vi "Image Name.vi"(8 "error in (no error)":errorcluster, 11 "CCDCamera in":refnum<class "CCDCamera.lvclass">) -> (0 "error out":errorcluster, 3 "CCDCamera out":refnum<class "CCDCamera.lvclass">)   [LabVIEW 2018, in "CCDCamera.lvclass"]
uses:
  CCDCamera.lvclass
  CCDCamera.lvclass/CCDCamera.ctl
  Interface/Interface.lvclass
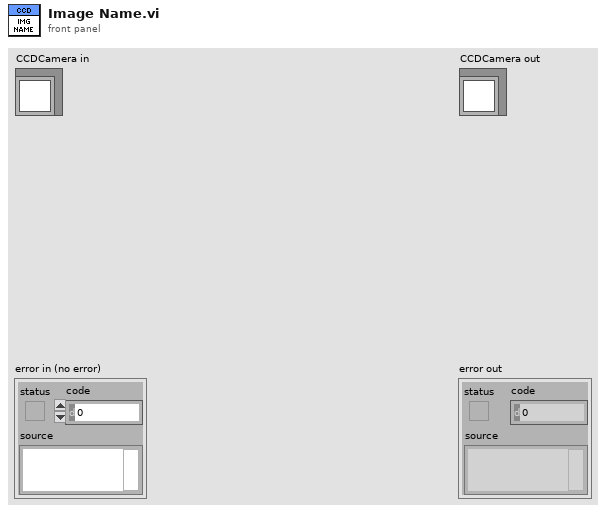
[diagram p1: front panel]
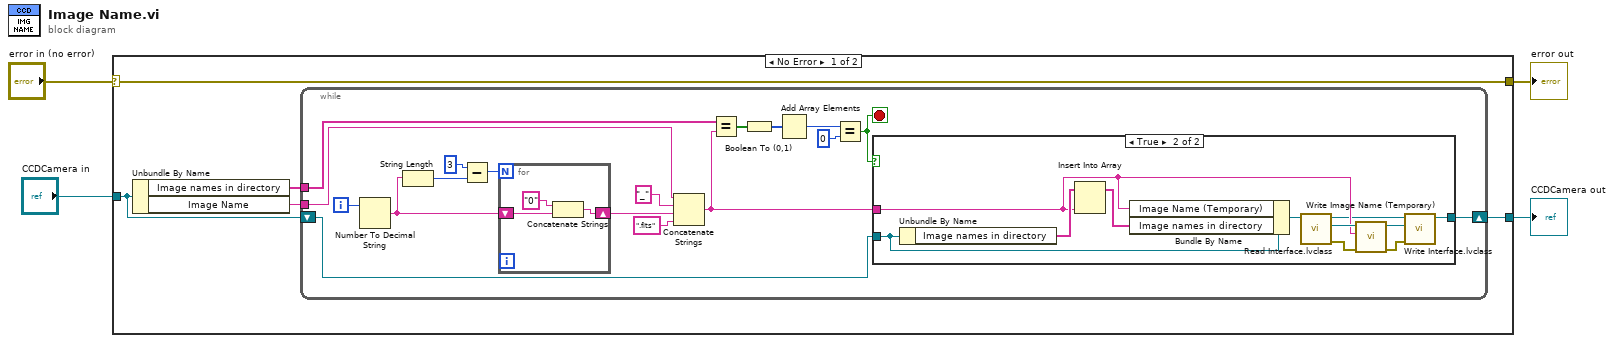
[diagram p0: block diagram]
diagram:
  n1 = case shown="No Error" "error in (no error)" {
    selector: "error in (no error)" -> [w9 w44]
    tunnel: [w9 w44] -> w3
    tunnel: [w7 w43] -> w1
    tunnel: "CCDCamera in" -> [w6 w43]
    frame No Error {
      n2 = Unbundle By Name(w6) -> ("Image names in directory"=w5:string[], "Image Name"=w8:string)
      n3 = while {
        tunnel: w5 -> [w27]
        tunnel: w8 -> [w19]
        shift-right: [w22] -> w7
        shift-left: w6 -> [w21]
        i -> [w20]
        stop <- w17 stop-if-true
        n4 = Number To Decimal String(number=w20) -> (decimal integer string=w10:string)  [unwired: 1 in]
        n5 = String Length(string=w10) -> (length=w13:i32)
        n6 = Subtract(x=3, y=w13) -> (x-y=w14:i32)
        n7 = for {
          N: w14 -> [_]
          shift-right: [w30] -> w11
          shift-left: w10 -> [w28]
          n8 = Concatenate Strings("0" ("string"), w28) -> (w30:string)
        }
        n9 = Concatenate Strings(w19, "_" ("string"), w11, ".fits" ("string")) -> (w18:string)
        n10 = Equal?(x=w27, y=w18) -> (x = y?=w26:bool[])
        n11 = Boolean To (0,1)(Boolean=w26) -> (0, 1=w25:i16[])
        n12 = Add Array Elements(numeric array=w25) -> (sum=w24:i16)
        n13 = Equal?(x=w24, y=0) -> (x = y?=w17:bool)
        n14 = case shown="True" w17 {
          tunnel: w18 -> [_ w33]
          tunnel: [w31 w37] -> w22
          tunnel: w21 -> [w31 w36]
          frame False {
          }
          frame True {
            n15 = Unbundle By Name(w36) -> ("Image names in directory"=w35:string[])
            n16 = Insert Into Array(array=w35, new element=w33) -> (w34:string[])  [unwired: 1 in]
            n17 = Bundle By Name(cluster=w36, "Image Name (Temporary)"=w33, "Image names in directory"=w34) -> (w38:refnum<class "CCDCamera.lvclass">)
            n18 = call-dynamic "Read Interface.lvclass.vi"("CCDCamera in"=w38) -> ("error out"=w41:errorcluster, "Interface.lvclass"=w40:refnum<class "Interface.lvclass">, "CCDCamera out"=w32:refnum<class "CCDCamera.lvclass">)  [unwired: 8 in]
            n19 = call-dynamic "Write Image Name (Temporary).vi"("error in (no error)"=w41, "Image Name (Temporary)"=w33, "Interface in"=w40) -> ("error out"=w42:errorcluster, "Interface out"=w39:refnum<class "Interface.lvclass">)  [unwired: 7 in]
            n20 = call-dynamic "Write Interface.lvclass.vi"("error in (no error)"=w42, "Interface.lvclass"=w39, "CCDCamera in"=w32) -> ("CCDCamera out"=w37:refnum<class "CCDCamera.lvclass">)  [unwired: 7 in, 1 out]
          }
        }
      }
    }
    frame Error {
    }
  }
  "error out" <- w3
  "CCDCamera out" <- w1
